vi "E441X_PM_Default_Inst_Setup.vi"(0 "VISA session":refnum<visa-resource-name>, 11 "error in (no error)":errorcluster) -> (4 "dup VISA session":refnum<visa-resource-name>, 15 "error out":errorcluster)   [LabVIEW 2015]
doc: "This Utility VI sends a default command string to the instrument whenever a new VISA session is opened, or the instrument is reset."
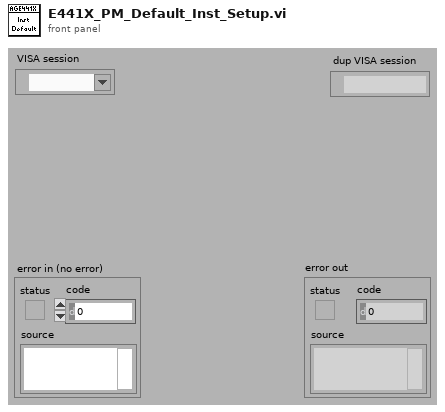
[diagram p1: front panel]
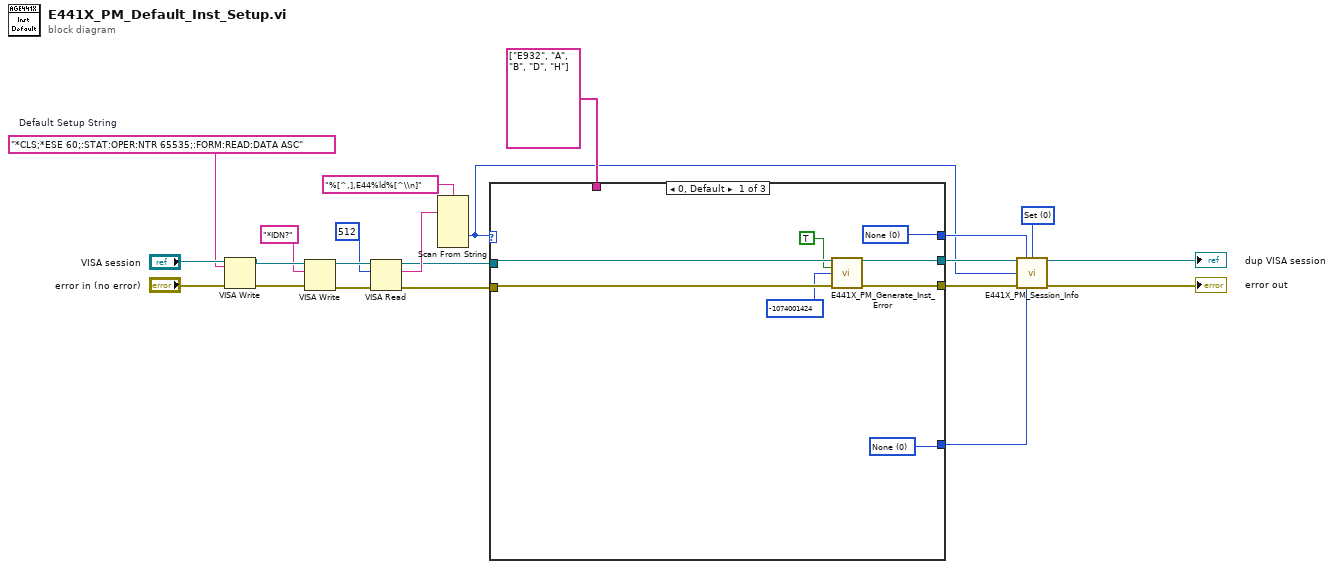
[diagram p0: block diagram]
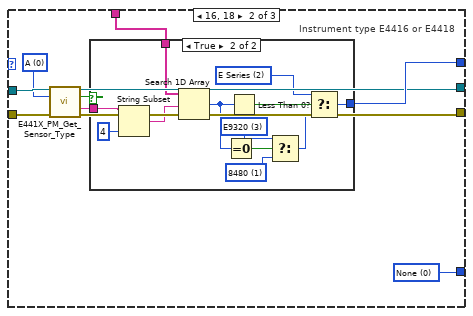
[diagram p2: hidden frame]
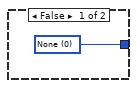
[diagram p3: hidden frame]
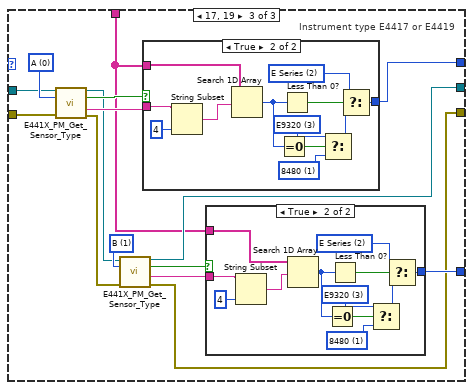
[diagram p4: hidden frame]
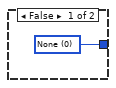
[diagram p5: hidden frame]
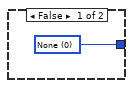
[diagram p6: hidden frame]
diagram:
  w5 = 0 items=["Set", "Get"] ("Operation")
  w20 = "*CLS;*ESE 60;:STAT:OPER:NTR 65535;:FORM:READ:DATA ASC"  # Default Setup String
  n1 = VISA Write(VISA resource name="VISA session", write buffer=w20, error in (no error)="error in (no error)") -> (VISA resource name out=w19:refnum<visa-resource-name>, error out=w18:errorcluster)  [unwired: 1 out]
  n2 = VISA Write(VISA resource name=w19, write buffer="*IDN?" ("Command"), error in (no error)=w18) -> (VISA resource name out=w16:refnum<visa-resource-name>, error out=w15:errorcluster)  [unwired: 1 out]
  n3 = VISA Read(VISA resource name=w16, byte count=u32 512 ("byte count (0)"), error in (no error)=w15) -> (VISA resource name out=w11:refnum<visa-resource-name>, read buffer=w13:string, error out=w10:errorcluster)  [unwired: 1 out]
  n4 = Scan From String(format string="%[^,],E44%ld%[^\\n]", input string=w13) -> (output 2=w4:i32)  [unwired: 7 in, 3 out]
  n5 = case shown="0, Default" w4 {
    tunnel: w11 -> [w26 w40 w67]
    tunnel: w10 -> [w25 w39 w66]
    tunnel: string[] ["E932", "A", "B", "D", "H"] -> [_ w35 w56]
    tunnel: [w30 w34 w63] -> w6
    tunnel: [w28 w32 w58] -> w8
    tunnel: [w29 w33 w55] -> w3
    tunnel: [w27 w31 w54] -> w7
    frame 0, Default {
      w29 = 0 items=["None", "8480", "E Series", "E9320"] ("Sensor B (0: None)")
      w30 = 0 items=["None", "8480", "E Series", "E9320"] ("Sensor B (0: None)")
      n6 = call "E441X_PM_Generate_Inst_Error.vi"("VISA session"=w26, "Error State (F: Off)"=TRUE, "Code (0 - No error)"=-1074001424, "error in (no error)"=w25) -> ("dup VISA session"=w28:refnum<visa-resource-name>, "error out"=w27:errorcluster)  [unwired: 10 in]
    }
    frame 16, 18 {
      w33 = 0 items=["None", "8480", "E Series", "E9320"] ("Sensor B (0: None)")
      w38 = 0 items=["A", "B"] ("Channel (0: A)")
      # "Instrument type E4416 or E4418"
      n7 = call "E441X_PM_Get_Sensor_Type.vi"("VISA session"=w40, "Channel (0: A)"=w38, "error in (no error)"=w39) -> ("dup VISA session"=w32:refnum<visa-resource-name>, "State"=w36:bool, "Sensor Type"=w37:string, "error out"=w31:errorcluster)  [unwired: 9 in]
      n8 = case shown="True" w36 {
        tunnel: w37 -> [_ w53]
        tunnel: w35 -> [_ w51]
        tunnel: [w41 w42] -> w34
        frame False {
          w41 = 0 items=["None", "8480", "E Series", "E9320"] ("Sensor B (0: None)")
        }
        frame True {
          w44 = 1 items=["None", "8480", "E Series", "E9320"] ("Sensor B (0: None)")
          w45 = 3 items=["None", "8480", "E Series", "E9320"] ("Sensor B (0: None)")
          w48 = 2 items=["None", "8480", "E Series", "E9320"] ("Sensor B (0: None)")
          n9 = String Subset(string=w53, length (rest)=4 ("length (rest)")) -> (substring=w50:string)  [unwired: 1 in]
          n10 = Search 1D Array(1D array=w51, element=w50) -> (index of element=w47:i32)  [unwired: 1 in]
          n11 = Equal To 0?(x=w47) -> (x = 0?=w46:bool)
          n12 = Less Than 0?(x=w47) -> (x < 0?=w49:bool)
          n13 = Select(t=w45, s=w46, f=w44) -> (s? t:f=w43:i32)
          n14 = Select(t=w48, s=w49, f=w43) -> (s? t:f=w42:i32)
        }
      }
    }
    frame 17, 19 {
      w61 = 1 items=["A", "B"] ("Channel (0: A)")
      w68 = 0 items=["A", "B"] ("Channel (0: A)")
      # "Instrument type E4417 or E4419"
      n15 = call "E441X_PM_Get_Sensor_Type.vi"("VISA session"=w67, "Channel (0: A)"=w68, "error in (no error)"=w66) -> ("dup VISA session"=w59:refnum<visa-resource-name>, "State"=w65:bool, "Sensor Type"=w64:string, "error out"=w60:errorcluster)  [unwired: 9 in]
      n16 = call "E441X_PM_Get_Sensor_Type.vi"("VISA session"=w59, "Channel (0: A)"=w61, "error in (no error)"=w60) -> ("dup VISA session"=w58:refnum<visa-resource-name>, "State"=w62:bool, "Sensor Type"=w57:string, "error out"=w54:errorcluster)  [unwired: 9 in]
      n17 = case shown="True" w65 {
        tunnel: w64 -> [_ w94]
        tunnel: w56 -> [_ w92]
        tunnel: [w82 w83] -> w63
        frame False {
          w82 = 0 items=["None", "8480", "E Series", "E9320"] ("Sensor B (0: None)")
        }
        frame True {
          w85 = 1 items=["None", "8480", "E Series", "E9320"] ("Sensor B (0: None)")
          w86 = 3 items=["None", "8480", "E Series", "E9320"] ("Sensor B (0: None)")
          w89 = 2 items=["None", "8480", "E Series", "E9320"] ("Sensor B (0: None)")
          n18 = String Subset(string=w94, length (rest)=4 ("length (rest)")) -> (substring=w91:string)  [unwired: 1 in]
          n19 = Search 1D Array(1D array=w92, element=w91) -> (index of element=w88:i32)  [unwired: 1 in]
          n20 = Equal To 0?(x=w88) -> (x = 0?=w87:bool)
          n21 = Less Than 0?(x=w88) -> (x < 0?=w90:bool)
          n22 = Select(t=w86, s=w87, f=w85) -> (s? t:f=w84:i32)
          n23 = Select(t=w89, s=w90, f=w84) -> (s? t:f=w83:i32)
        }
      }
      n24 = case shown="True" w62 {
        tunnel: w57 -> [_ w81]
        tunnel: w56 -> [_ w79]
        tunnel: [w69 w70] -> w55
        frame False {
          w69 = 0 items=["None", "8480", "E Series", "E9320"] ("Sensor B (0: None)")
        }
        frame True {
          w72 = 1 items=["None", "8480", "E Series", "E9320"] ("Sensor B (0: None)")
          w73 = 3 items=["None", "8480", "E Series", "E9320"] ("Sensor B (0: None)")
          w76 = 2 items=["None", "8480", "E Series", "E9320"] ("Sensor B (0: None)")
          n25 = String Subset(string=w81, length (rest)=4 ("length (rest)")) -> (substring=w78:string)  [unwired: 1 in]
          n26 = Search 1D Array(1D array=w79, element=w78) -> (index of element=w75:i32)  [unwired: 1 in]
          n27 = Equal To 0?(x=w75) -> (x = 0?=w74:bool)
          n28 = Less Than 0?(x=w75) -> (x < 0?=w77:bool)
          n29 = Select(t=w73, s=w74, f=w72) -> (s? t:f=w71:i32)
          n30 = Select(t=w76, s=w77, f=w71) -> (s? t:f=w70:i32)
        }
      }
    }
  }
  n31 = call "E441X_PM_Session_Info.vi"("VISA session"=w8, "Sensor A (0:None)"=w6, "Operation"=w5, "Instrument Number (16)"=w4, "error in (no error)"=w7, "Sensor B (0:None)"=w3) -> ("dup VISA session"=→"dup VISA session":refnum<visa-resource-name>, "error out"=→"error out":errorcluster)  [unwired: 4 in, 4 out]
